vi "exp2.vi"() -> ()   [LabVIEW 2014]
uses:
  <vilib>/DAQmx/create/channels.llb/DAQmx Create Channel (AO-Voltage-Basic).vi
  <vilib>/DAQmx/write.llb/DAQmx Write (Analog DBL 1Chan 1Samp).vi
  <vilib>/DAQmx/create/channels.llb/DAQmx Create Channel (AI-Voltage-Basic).vi
  <vilib>/DAQmx/read.llb/DAQmx Read (Analog DBL 1Chan 1Samp).vi
panel:
  in  "停止测量":bool
  in  "输入通道":tag
  out "测量电压":dbl
  in  "输出电压":dbl
  in  "停止输出":bool
  in  "输出通道":tag
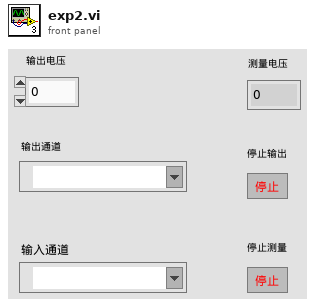
[diagram p1: front panel]
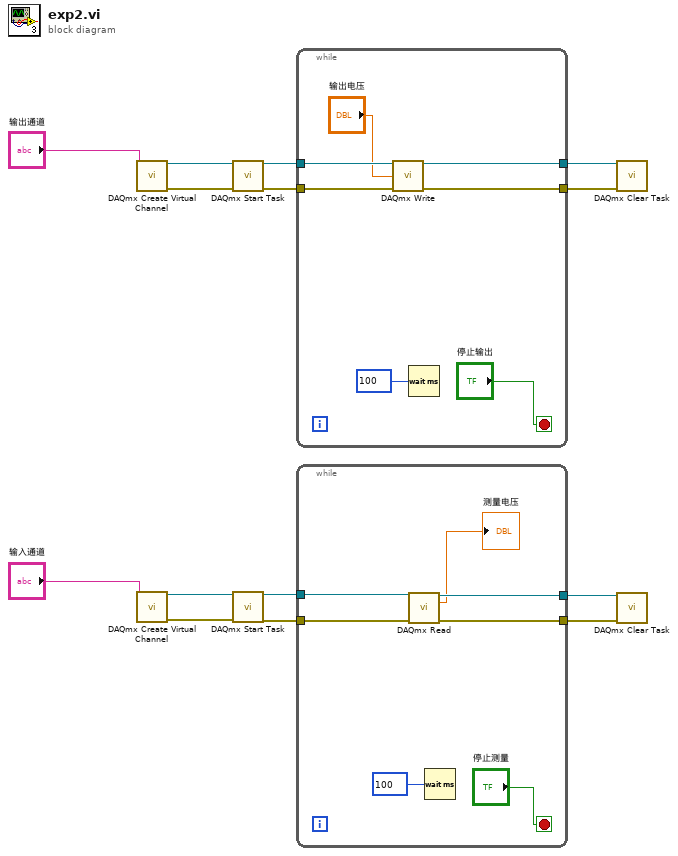
[diagram p0: block diagram]
diagram:
  n1 = call-poly <vilib>:"DAQmx Create Virtual Channel.vi"("physical channels"="输出通道") -> ("task out"=w12:refnum<k21>, "error out"=w7:errorcluster)  [unwired: 13 in]
  n2 = call-poly <vilib>:"DAQmx Create Virtual Channel.vi"("physical channels"="输入通道") -> ("task out"=w6:refnum<k21>, "error out"=w5:errorcluster)  [unwired: 13 in]
  n3 = call <vilib>:"DAQmx Start Task.vi"("task/channels in"=w12, "error in"=w7) -> ("task out"=w11:refnum<k21>, "error out"=w8:errorcluster)  [unwired: 12 in]
  n4 = call <vilib>:"DAQmx Start Task.vi"("task/channels in"=w6, "error in"=w5) -> ("task out"=w4:refnum<k21>, "error out"=w1:errorcluster)  [unwired: 12 in]
  n5 = while {
    tunnel: w11 -> [w19]
    tunnel: [w18] -> w10
    tunnel: [w17] -> w9
    tunnel: w8 -> [w16]
    stop <- "停止输出" stop-if-true
    n6 = call-poly <vilib>:"DAQmx Write.vi"("task/channels in"=w19, "data"="输出电压", "error in"=w16) -> ("task out"=w18:refnum<k21>, "error out"=w17:errorcluster)  [unwired: 10 in, 1 out]
    n7 = Wait (ms)(milliseconds to wait=u32 100 ("等待时间（毫秒）")) -> ()  [unwired: 1 out]
  }
  n8 = while {
    tunnel: w4 -> [w26]
    tunnel: [w25] -> w3
    tunnel: [w24] -> w2
    tunnel: w1 -> [w23]
    stop <- "停止测量" stop-if-true
    n9 = call-poly <vilib>:"DAQmx Read.vi"("task/channels in"=w26, "error in"=w23) -> ("task out"=w25:refnum<k21>, "data"=→"测量电压":dbl, "error out"=w24:errorcluster)  [unwired: 11 in]
    n10 = Wait (ms)(milliseconds to wait=u32 100 ("等待时间（毫秒）")) -> ()  [unwired: 1 out]
  }
  n11 = call <vilib>:"DAQmx Clear Task.vi"("task in"=w10, "error in"=w9) -> ()  [unwired: 13 in, 1 out]
  n12 = call <vilib>:"DAQmx Clear Task.vi"("task in"=w3, "error in"=w2) -> ()  [unwired: 13 in, 1 out]
